vi "Image_Display_RAW12_U8.vi"(7 "Bayer Pattern":T2, 8 "error in (no error)":errorcluster, 9 "Image Name":string="RAW12_U8", 10 "Image Configuration":T1={"Width"=3840, "Height"=2160}, 11 "RAW12 Frame (U8)":u8[](array[numeric])) -> (0 "error out":errorcluster, 1 "Image":T3(plugin-control), 2 "Image Configuration Out":T1={"Width"=3840, "Height"=2160}, 3 "RGB Frame Out":u8[](array[numeric]))   [LabVIEW 2020]
uses:
  ctl/Image_Configuration.ctl
  ctl/Image_RAW_Bayer_Pattern.ctl
  <vilib>/vision/Image Controls.llb/IMAQ Image.ctl
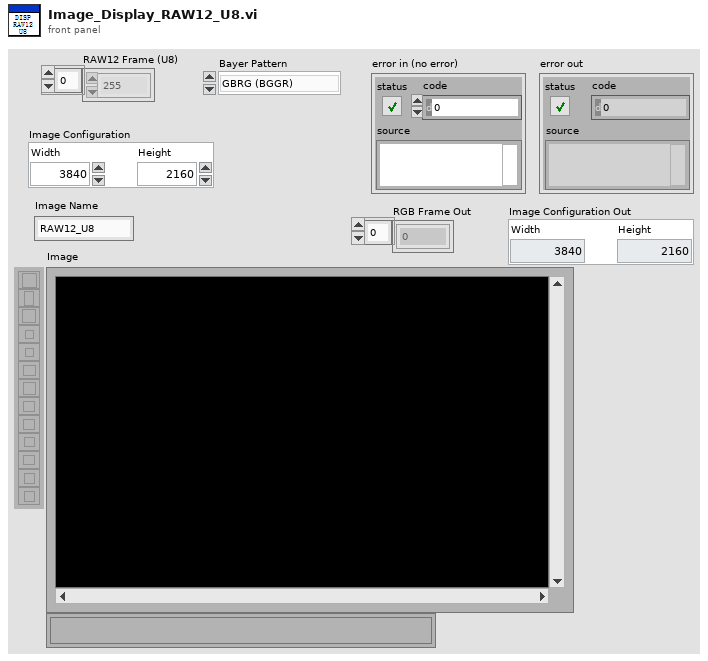
[diagram p1: front panel]
types:
  T1 = typedef "Image_Configuration.ctl" = cluster{"Width":i32, "Height":i32}
  T2 = typedef "Image_RAW_Bayer_Pattern.ctl" = enum16{"GBRG (BGGR)", "GRBG (RGGB)", "BGGR (GBRG)", "RGGB (GRBG)", "CRBC (RCCB)"}
  T3 = typedef "IMAQ Image.ctl" = refnum<image>
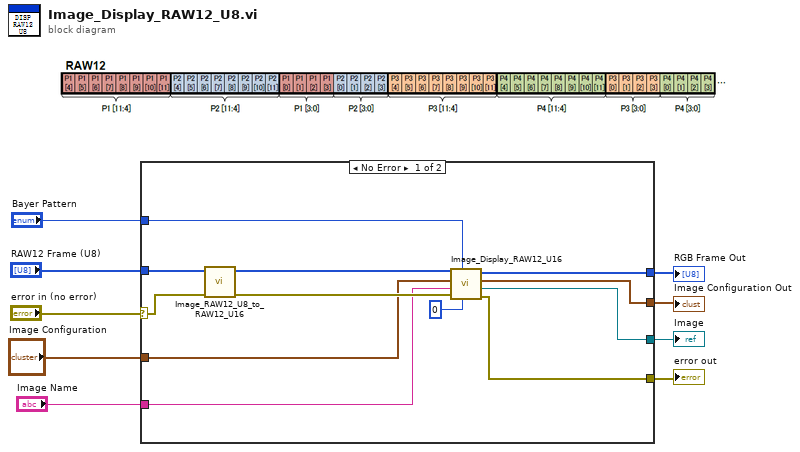
[diagram p0: block diagram]
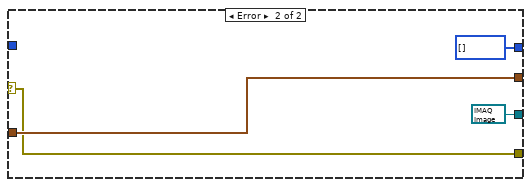
[diagram p2: hidden frame]
diagram:
  n1 = case shown="No Error" "error in (no error)" {
    selector: "error in (no error)" -> [w20 w22]
    tunnel: "Image Configuration" -> [w16 w24]
    tunnel: "RAW12 Frame (U8)" -> [w21 _]
    tunnel: "Bayer Pattern" -> [w17 _]
    tunnel: "Image Name" -> [w15 _]
    tunnel: [w14 u8[] [] ("RGB Frame Out")] -> w4
    tunnel: [w13 w24] -> w3
    tunnel: [w12 T3 refnum ("Image")] -> w2
    tunnel: [w11 w22] -> w1
    frame No Error {
      n2 = call "Image_RAW12_U8_to_RAW12_U16.vi"("error in (no error)"=w20, "RAW12 Frame (U8)"=w21) -> ("error out"=w18:errorcluster, "RAW12 Frame (U16)"=w19:u16[])  [unwired: 8 in]
      n3 = call "Image_Display_RAW12_U16.vi"("Scale by Power of 2"=i16 0, "Bayer Pattern"=w17, "error in (no error)"=w18, "Image Name"=w15, "Image Configuration"=w16, "RAW12_U16"=w19) -> ("error out"=w11:errorcluster, "Image"=w12:T3, "Image Configuration Out"=w13:T1, "RGB Frame Out"=w14:u8[])  [unwired: 2 in]
    }
    frame Error {
    }
  }
  "error out" <- w1
  "Image" <- w2
  "RGB Frame Out" <- w4
  "Image Configuration Out" <- w3
